vi "WriteFalconProcessed.vi"(0 "Path:~\\syslogs\\FalconProcessed":path, 7 "FalconProcessedData":u8[](array[numeric])=array[44904 elements]) -> (15 "error out":errorcluster)   [LabVIEW 2011]
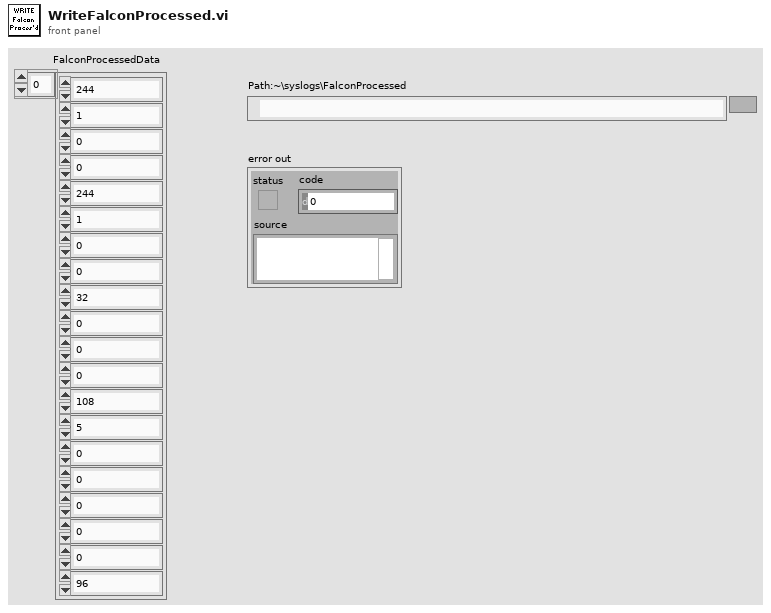
[diagram p1: front panel]
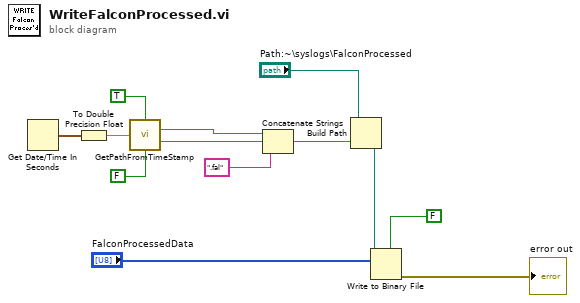
[diagram p0: block diagram]
diagram:
  n1 = Get Date/Time In Seconds() -> (seconds since 1Jan1904=w13:timestamp)
  n2 = To Double Precision Float(number=w13) -> (double precision float=w12:dbl)
  n3 = call "GetPathFromTimeStamp.vi"("UTC Time"=TRUE, "LocalTimeStamp"=w12, "Changement de date à midi ?"=FALSE) -> ("Date String"=w11:string, "Time String"=w10:string)  [unwired: 11 in]
  n4 = Concatenate Strings(w11, w10, ".fal") -> (w8:string)
  n5 = Build Path(base path="Path:~\\syslogs\\FalconProcessed", name or relative path=w8) -> (appended path=w6:path)
  n6 = Write to Binary File(file (use dialog)=w6, data="FalconProcessedData", 5:FALSE ("prepend array or string size? (T)")) -> (error out=→"error out":errorcluster)  [unwired: 3 in, 2 out]
